vi "GetNumeric.vi"(10 "B":i32=777, 11 "A":i32=777) -> (3 "Numeric Out":i32=777)   [LabVIEW 2017]
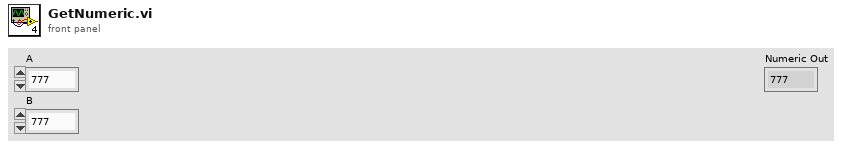
[diagram p1: front panel]
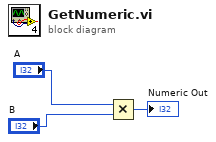
[diagram p0: block diagram]
diagram:
  n1 = Multiply(x="A", y="B") -> (x*y=→"Numeric Out":i32)
